vi "bodyTest.vi"(7 "LabVIEW Web Service Request":refnum<class "Web Request.lvclass">, 10 "nominalPressure":dbl caption="pressure" format="%#g", 11 "time":dbl format="%#g") -> (2 "value":string, 3 "actualPressure":dbl)   [LabVIEW 2015]
uses:
  <vilib>/wsapi/Web Request.lvclass
  <vilib>/Waveform/WDTOps.llb/WDT Append Waveforms DBL.vi
panel:
  in  "Start timer":bool
  out "data":waveform(dbl)[](graph)
  out "timer":dbl
  in  "Stop timer":bool
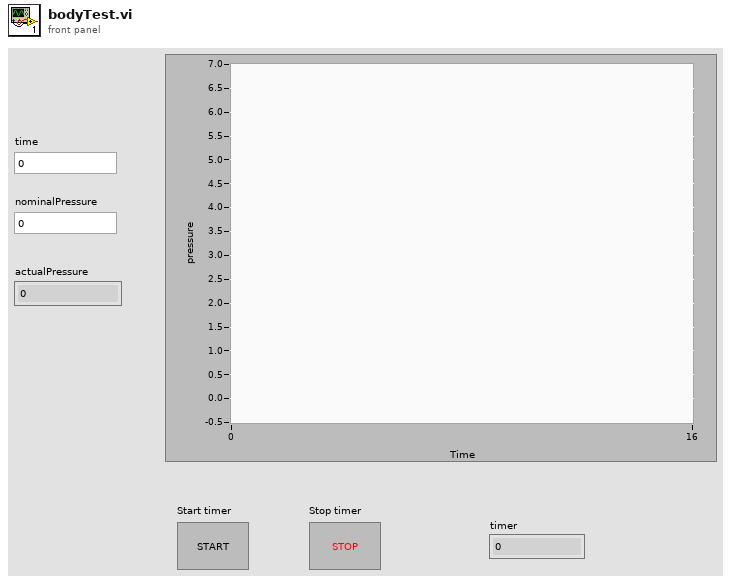
[diagram p1: front panel]
types:
  T1 = typedef "imagedata.ctl" = cluster{"image type":i32, "image depth":i32, "image":u8[], "mask":u8[], "colors":u32[], "Rectangle":cluster{"left":i16, "top":i16, "right":i16, "bottom":i16}}
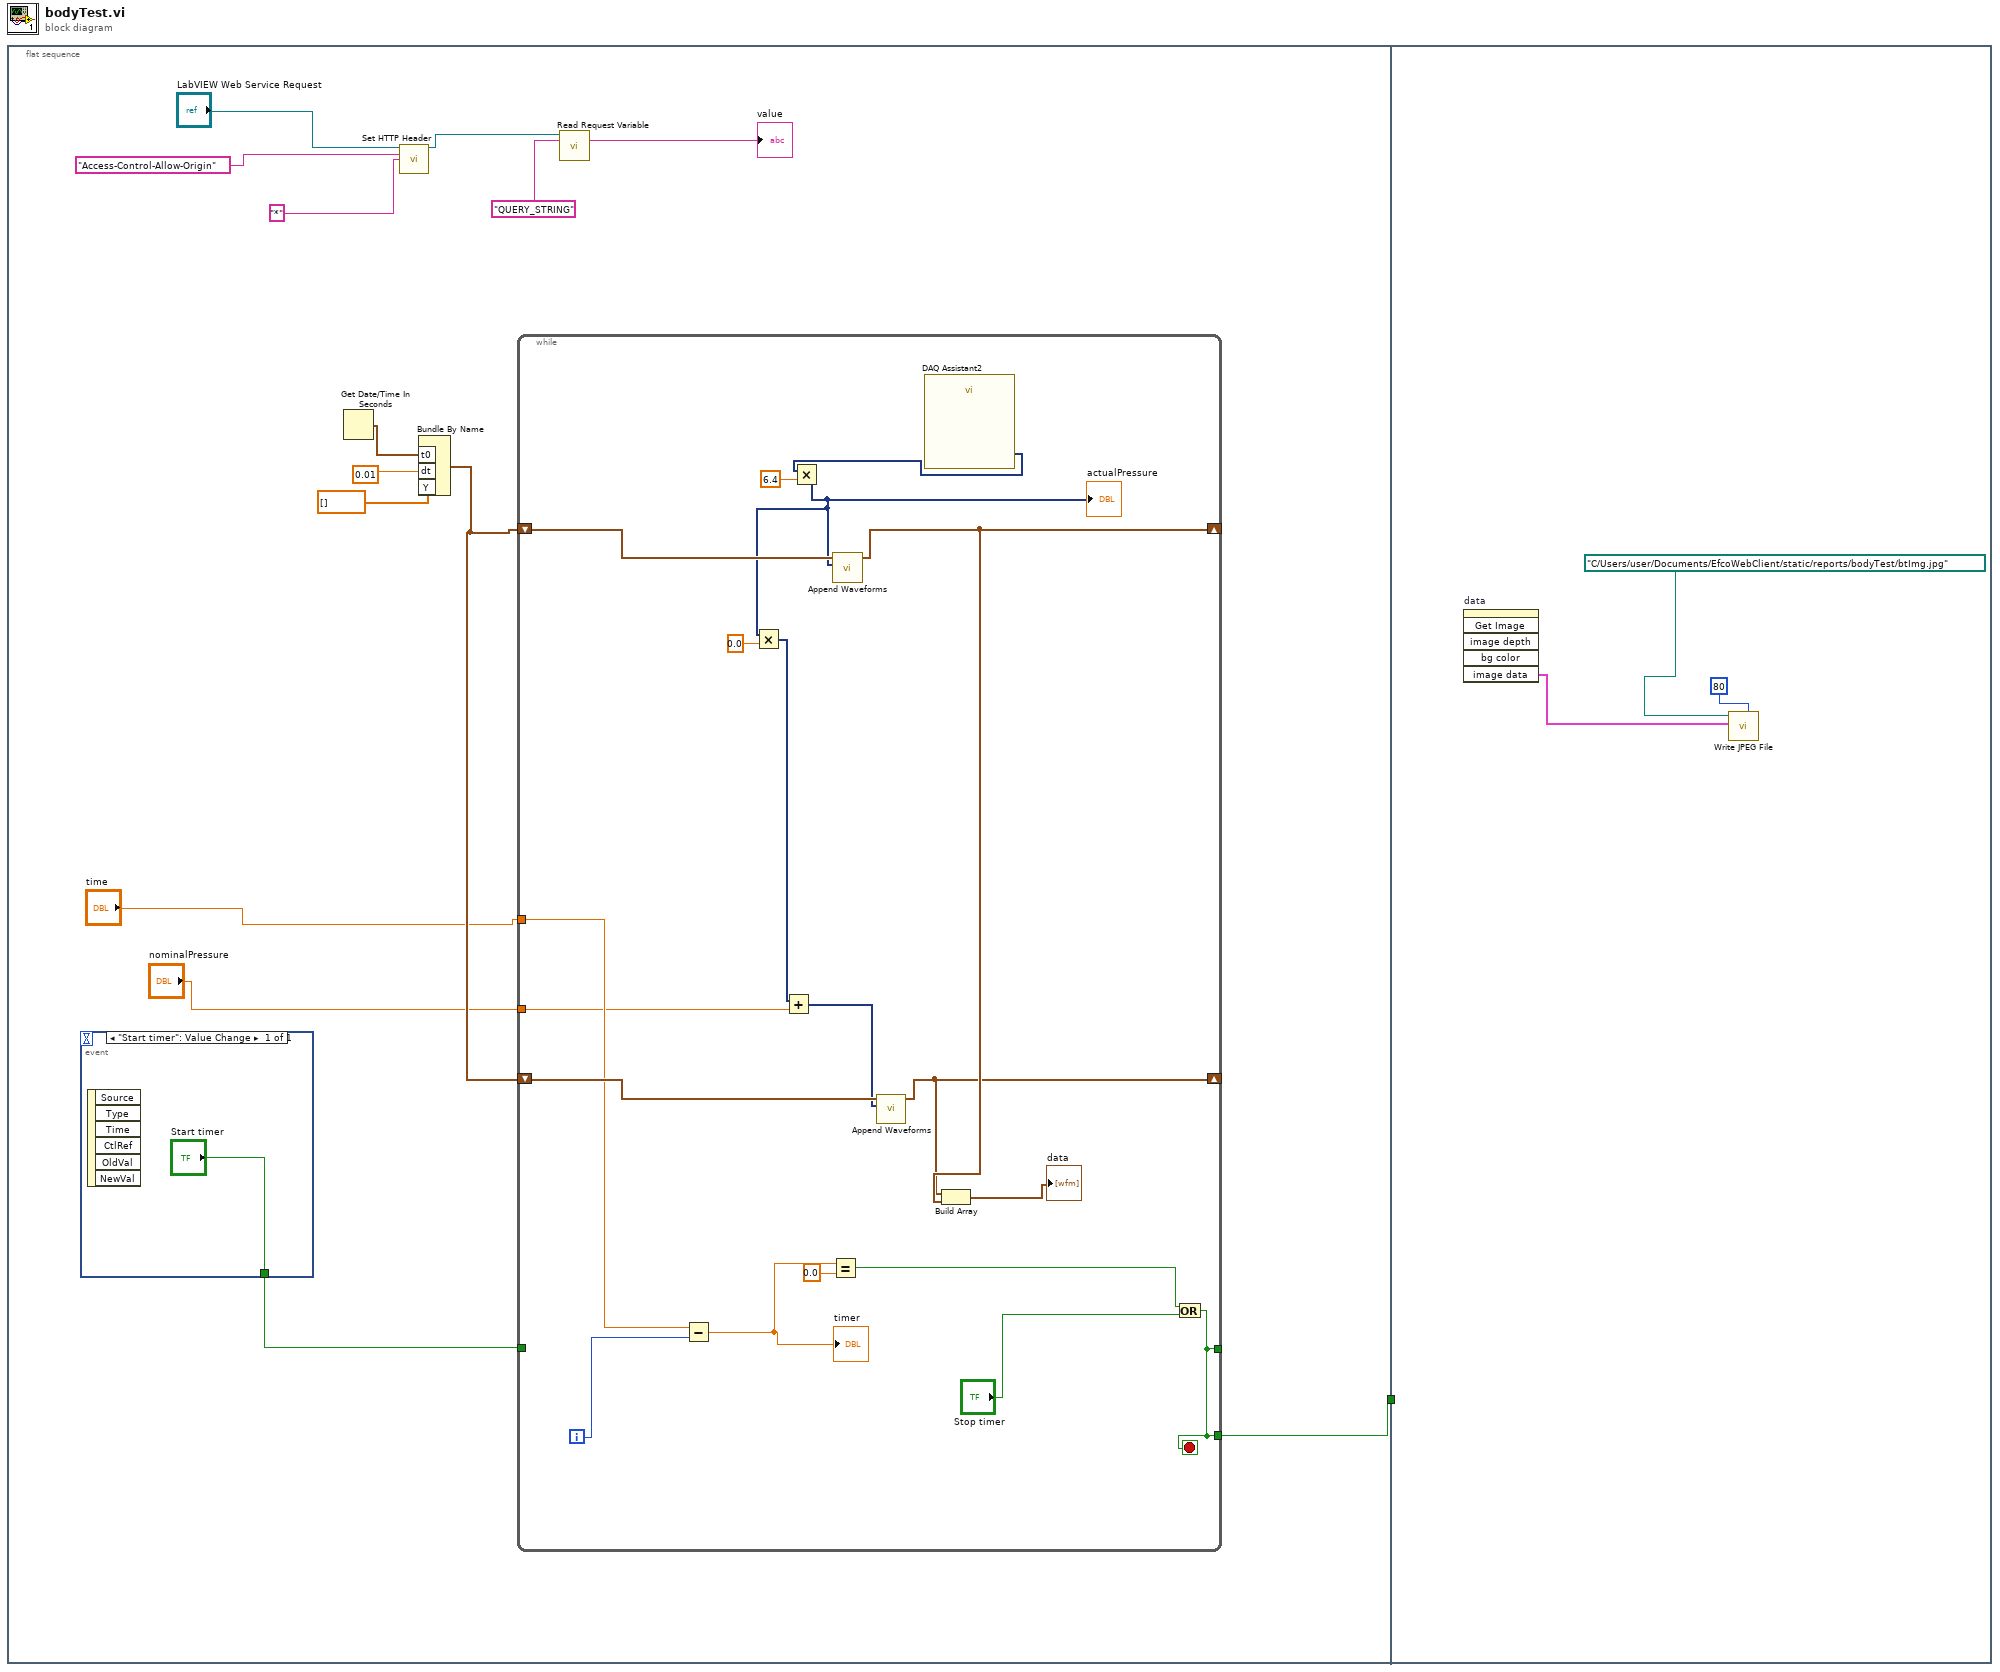
[diagram p0: block diagram]
diagram:
  n1 = flat-sequence {
    tunnel: [w8] -> w1
    tunnel: w1 -> [_]
    frame #0 {
      n2 = event shown="[0] \"Start timer\": Value Change" {
        selector: _ -> [_]
        dyn-events: _ -> [_]
        timeout: _ -> [_]
        tunnel: ["Start timer"] -> w12
        event "Start timer": Value Change {
          n3 = event-data() -> ()  [unwired: 1 in, 6 out]
        }
      }
      n4 = Get Date/Time In Seconds() -> (seconds since 1Jan1904=w15:timestamp)
      n5 = call <vilib>:"Set HTTP Header.vi"("LabVIEW Web Service Request"="LabVIEW Web Service Request", "header"="Access-Control-Allow-Origin", "header value"="*") -> ("LabVIEW Web Service Request out"=w4:refnum<class "Web Request.lvclass">)  [unwired: 11 in, 1 out]
      n6 = Bundle By Name("t0"=w15, "dt"=0.01, "Y"=dbl[] []) -> (w11:waveform(dbl))  [unwired: 1 in]
      n7 = while {
        shift-right: [w29] -> _
        shift-left: w11 -> [w35]
        tunnel: "time" -> [w24]
        shift-right: [w28] -> _
        shift-left: w11 -> [w33]
        tunnel: w12 -> [_]
        tunnel: "nominalPressure" -> [w18]
        tunnel: [w17] -> _
        tunnel: [w17] -> w8
        i -> [w25]
        stop <- w17 stop-if-true
        n8 = Subtract(x=w24, y=w25) -> (x-y=w23:dbl)
        "timer" <- w23
        n9 = Equal?(x=w23, y=0.0) -> (x = y?=w21:bool)
        n10 = call "DAQ Assistant2"() -> ("data"=w27:dynamicdata)  [unwired: 16 in, 3 out]
        n11 = Multiply(x=w27, y=6.4) -> (x*y=w32:dynamicdata)
        "actualPressure" <- w32
        n12 = Multiply(x=w32, y=0.0) -> (x*y=w30:dynamicdata)
        n13 = Add(x=w30, y=w18) -> (x+y=w19:dynamicdata)
        n14 = call-poly <vilib>:"Append Waveforms.vi"("waveform B"=w32, "waveform A"=w35) -> ("waveform out"=w29:waveform(dbl))  [unwired: 8 in, 1 out]
        n15 = call-poly <vilib>:"Append Waveforms.vi"("waveform B"=w19, "waveform A"=w33) -> ("waveform out"=w28:waveform(dbl))  [unwired: 8 in, 1 out]
        n16 = Build Array(w28, w29) -> (→"data":waveform(dbl)[])
        n17 = Or(x=w21, y="Stop timer") -> (x .or. y?=w17:bool)
      }
      n18 = call <vilib>:"Read Request Variable.vi"("LabVIEW Web Service Request"=w4, "variable name"="QUERY_STRING") -> ("value"=→"value":string)  [unwired: 11 in, 2 out]
    }
    frame #1 {
      n19 = invoke on="data" class="WFGraph (strict)" method="Get Image"() -> ("image data"=w36:T1)  [unwired: 6 in, 5 out]
      n20 = call <vilib>:"Write JPEG File.vi"("quality (80)"=80, "image data"=w36, "path to JPEG file"=path "C:/Users/user/Documents/EfcoWebClient/static/reports/bodyTest/btImg.jpg") -> ()  [unwired: 7 in, 2 out]
    }
  }
